vi "Init Report.vi"(8 "error in (no error)":errorcluster, 11 "ResultProcessor Config in":refnum<class "ResultProcessor Config.lvclass">) -> (0 "error out":errorcluster, 2 "Report.lvclass":refnum<class "Report.lvclass">, 3 "ResultProcessor Config out":refnum<class "ResultProcessor Config.lvclass">)   [LabVIEW 2015, in "ResultProcessor Config.lvclass"]
doc: "This VI returns a Report runtime class using the given configuration."
uses:
  ResultProcessor Config.lvclass
  Report/Generic/Execution/Report.lvclass
  ResultProcessor Config.lvclass/ResultProcessor Config.ctl
  Report/Generic/Config/Report Config.lvclass
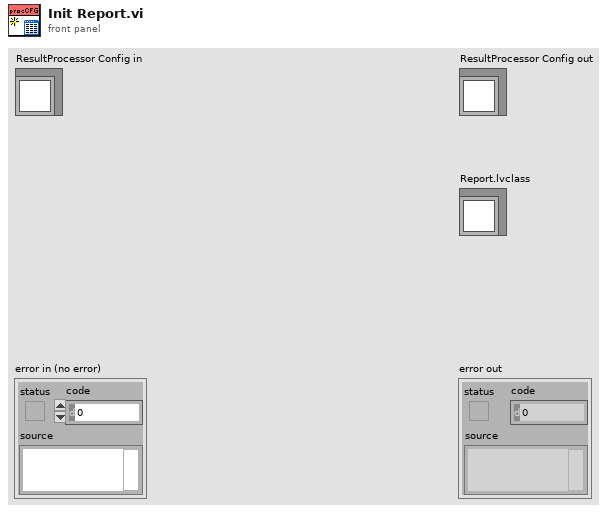
[diagram p1: front panel]
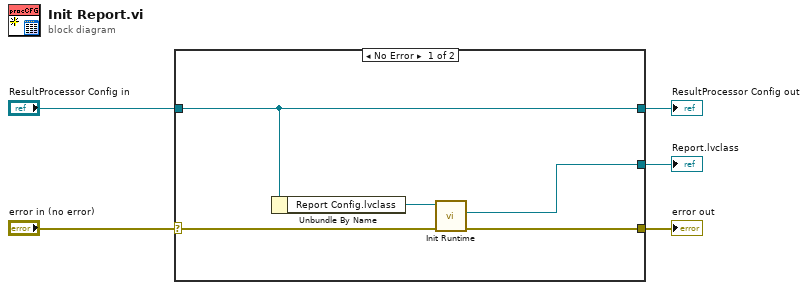
[diagram p0: block diagram]
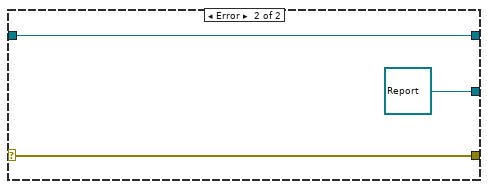
[diagram p2: hidden frame]
diagram:
  n1 = case shown="No Error" "error in (no error)" {
    selector: "error in (no error)" -> [w8 w13]
    tunnel: [w7 w13] -> w4
    tunnel: [w10 w12] -> w2
    tunnel: "ResultProcessor Config in" -> [w10 w12]
    tunnel: [w6 refnum<class "Report.lvclass"> refnum ("Report.lvclass")] -> w1
    frame No Error {
      n2 = Unbundle By Name(w10) -> ("Report Config.lvclass"=w9:refnum<class "Report Config.lvclass">)
      n3 = call-dynamic "Init Runtime.vi"("error in (no error)"=w8, "Report Config in"=w9) -> ("error out"=w7:errorcluster, "Report.lvclass"=w6:refnum<class "Report.lvclass">)  [unwired: 7 in, 1 out]
    }
    frame Error {
    }
  }
  "error out" <- w4
  "ResultProcessor Config out" <- w2
  "Report.lvclass" <- w1
